vi "Acquisition Message Loop.vi"(8 "error in (no error)":errorcluster, 11 "Message Queues":T2) -> (0 "error out":errorcluster)   [LabVIEW 2024, in "Acquisition.lvlib"]
doc: "Message loop for handling messages pertaining to the acquisition of data from the hardware."
uses:
  Acquisition.lvlib
  <vilib>/Utility/error.llb/Error Cluster From Error Code.vi
  Hardware Configuration.ctl
  support/Message Queue/Message Queue.lvlib
  support/Message Queue/Enqueue Message (Single).vi
  <vilib>/ErrorRing/Error Ring.xnode
  Acquisition State.ctl
  support/Message Queue/Enqueue Message (Array).vi
  support/Message Queue/Message Cluster.ctl
  support/Message Queue/All Message Queues.ctl
  controls/dataRefs.ctl
panel:
  in  "dataRef":T1
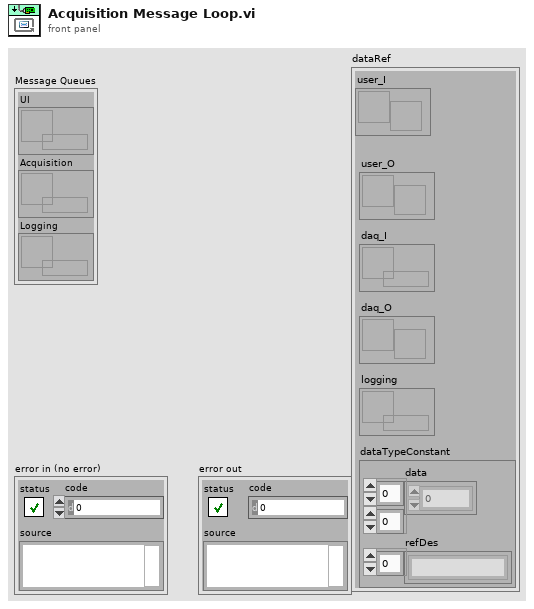
[diagram p1: front panel]
types:
  T1 = typedef "dataRefs.ctl" = cluster{"dataTypeConstant":cluster{"data":dbl[][], "refDes":string[]}, "user_I":refnum<notifier>, "user_O":refnum<notifier>, "daq_O":refnum<notifier>, "logging":refnum<queue>, "daq_I":refnum<queue>}
  T2 = typedef "Message Queue.lvlib/All Message Queues.ctl" = cluster{"UI":refnum<queue>, "Acquisition":refnum<queue>, "Logging":refnum<queue>}
  T3 = typedef "Acquisition.lvlib/Hardware Configuration.ctl" = cluster{"AI":cluster{"DAQmx Channel":tag, "Max Input":dbl, "Min Input":dbl, "Sample Rate":dbl, "DAQmx Task":refnum<k21>, "shunt resistor location":i32, "external shunt resistor value":dbl}, "AO":cluster{"DAQmx Channel":tag, "Max Output":dbl, "Min Output":dbl, "Sample Rate":dbl, "DAQmx Task":refnum<k21>}, "DO":cluster{"DAQmx Channel":tag, "Sample Rate":dbl, "DAQmx Task":refnum<k21>}, "DI":cluster{"DAQmx Channel":tag, "Sample Rate":dbl, "DAQmx Task":refnum<k21>}, "TC":cluster{"DAQmx Channel":tag, "Max Inout":dbl, "Min Input":dbl, "Sample Rate":dbl, "DAQmx Task":refnum<k21>, "resistance configuration":i32, "r0":dbl, "current excitation value":dbl, "current excitation source":i32, "rtd type":i32}}
  T4 = typedef "Acquisition.lvlib/Acquisition State.ctl" = enum16{"Idle", "Acquiring"}
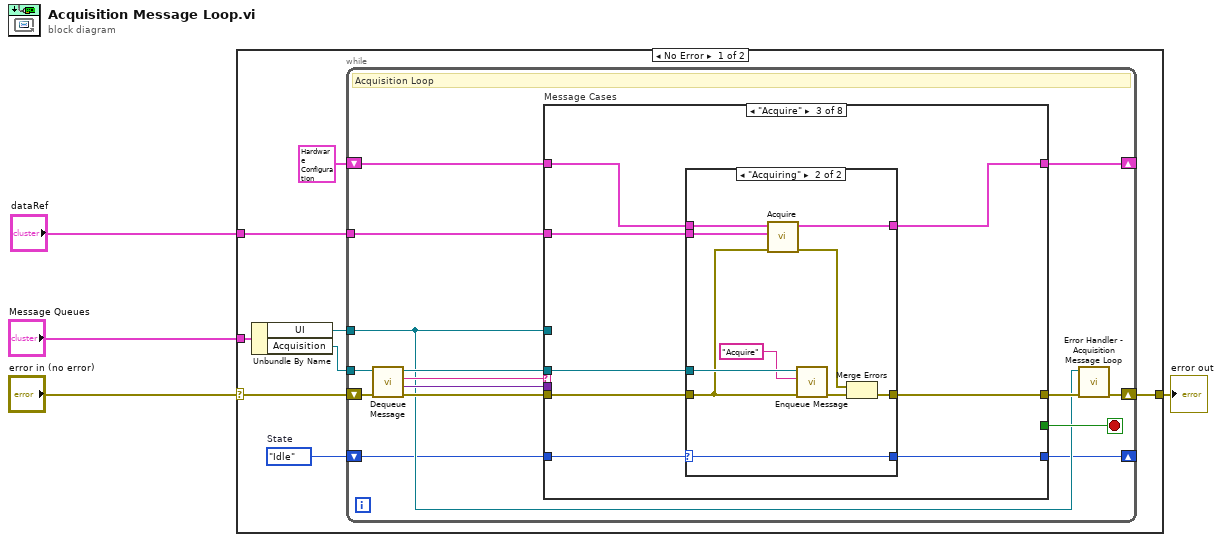
[diagram p0: block diagram]
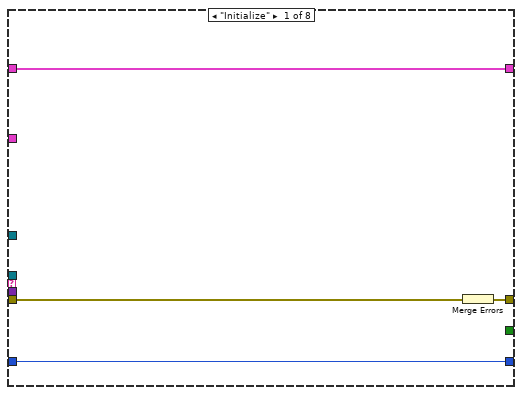
[diagram p2: hidden frame]
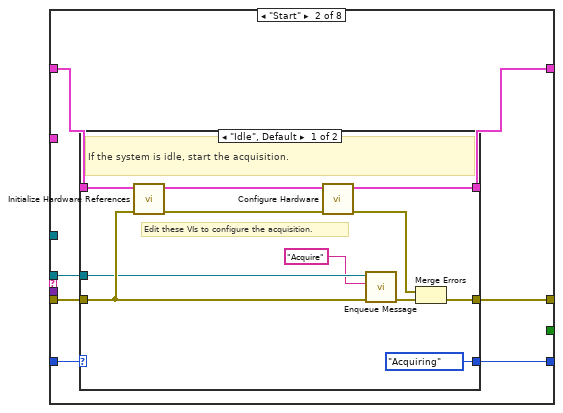
[diagram p3: hidden frame]
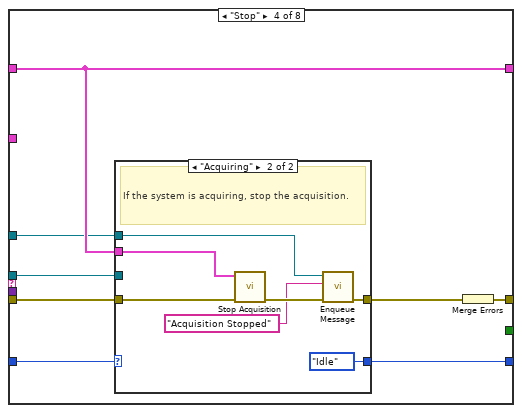
[diagram p6: hidden frame]
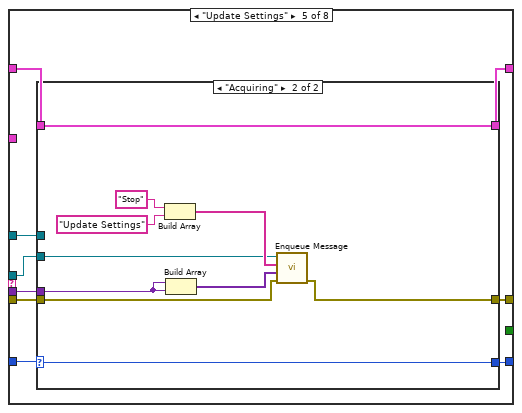
[diagram p8: hidden frame]
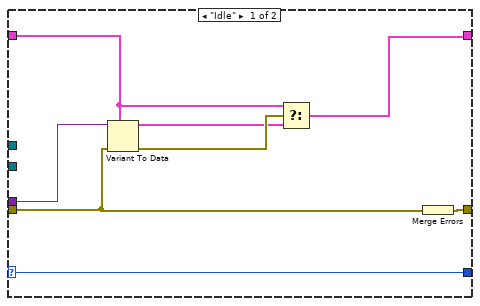
[diagram p9: hidden frame]
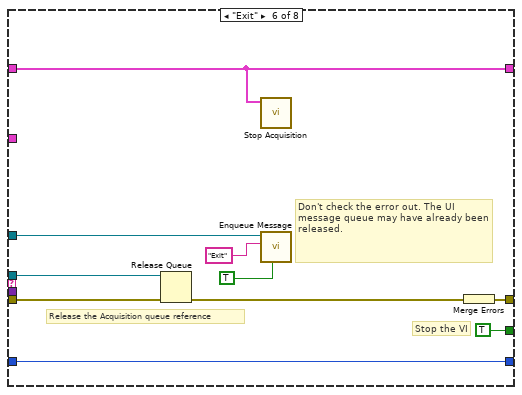
[diagram p10: hidden frame]
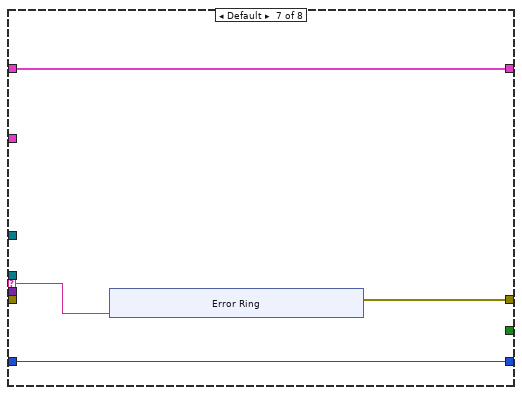
[diagram p11: hidden frame]
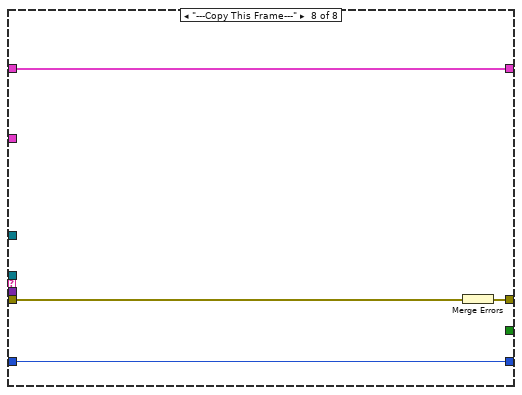
[diagram p12: hidden frame]
diagram:
  n1 = case shown="No Error" "error in (no error)" {
    selector: "error in (no error)" -> [w8 w143]
    tunnel: "Message Queues" -> [w12 _]
    tunnel: [w10 w143] -> w3
    tunnel: "dataRef" -> [w5 _]
    frame No Error {
      w6 = Acquisition_State."Idle"  # State
      n2 = Unbundle By Name(w12) -> ("UI"=w7:refnum<queue>, "Acquisition"=w11:refnum<queue>)
      n3 = while {
        tunnel: w11 -> [w19]
        shift-right: [w26] -> _
        shift-left: T3 {"AI"={"DAQmx Channel"="", "Max Input"=0.0, "Min Input"=0.0, "Sample Rate"=0.0, "DAQmx Task"="", "shunt resistor location"=-1, "external shunt resistor value"=249.0}, "AO"={"DAQmx Channel"="", "Max Output"=0.0, "Min Output"=0.0, "Sample Rate"=0.0, "DAQmx Task"=""}, "DO"={"DAQmx Channel"="", "Sample Rate"=0.0, "DAQmx Task"=""}, "DI"={"DAQmx Channel"="", "Sample Rate"=0.0, "DAQmx Task"=""}, "TC"={"DAQmx Channel"="", "Max Inout"=0.0, "Min Input"=0.0, "Sample Rate"=0.0, "DAQmx Task"="", "resistance configuration"=4, "r0"=100.0, "current excitation value"=0.0025, "current excitation source"=10167, "rtd type"=12481}} ("Data Cluster") -> [w27]
        shift-right: [w17] -> w10
        shift-left: w8 -> [w24]
        tunnel: w7 -> [w16]
        shift-right: [w14] -> _
        shift-left: w6 -> [w15]
        tunnel: w5 -> [w13]
        stop <- w25 stop-if-true
        # "Acquisition Loop"
        n4 = call "Dequeue Message.vi"("error in (no error)"=w24, "Message Queue"=w19) -> ("error out"=w23:errorcluster, "Message Data"=w21:variant, "Message"=w22:string, "dup Message Queue"=w20:refnum<queue>)  [unwired: 6 in]
        n5 = case "Message Cases" shown="\"Acquire\"" w22 {
          selector: w22 -> [_ _ _ _ _ _ w130 _]
          tunnel: w20 -> [_ w35 w59 w78 w91 w120 _ _]
          tunnel: w23 -> [w30 w36 w58 w80 w95 w124 _ w142]
          tunnel: [w31 w38 w60 w81 w99 w126 w129 w140] -> w18
          tunnel: w27 -> [w29 w37 w56 w79 w97 w119 w131 w141]
          tunnel: [w29 w34 w57 w79 w96 w119 w131 w141] -> w26
          tunnel: [_ _ _ _ _ TRUE _ _] -> w25
          tunnel: w21 -> [_ _ _ _ w98 _ _ _]
          tunnel: w16 -> [_ _ _ w77 w92 w125 _ _]
          tunnel: w15 -> [w28 w33 w55 w76 w94 w118 w128 w139]
          tunnel: [w28 w32 w54 w75 w93 w118 w128 w139] -> w14
          tunnel: w13 -> [_ _ w53 _ _ _ _ _]
          frame "Initialize" {
            # "Initialize  - Initialize is currently a no-op.  The hardware initialization takes place in the 'Start' message."
            n6 = Merge Errors(w30) -> (w31:errorcluster)
          }
          frame "Start" {
            # "Start - Configure and start the acquisition."
            n7 = case shown="\"Idle\", Default" w33 {
              selector: w33 -> [_ w50]
              tunnel: [w49 w52] -> w38
              tunnel: w37 -> [w48 w51]
              tunnel: w36 -> [w47 w52]
              tunnel: w35 -> [w45 _]
              tunnel: [w41 w51] -> w34
              tunnel: [Acquisition_State."Acquiring" ("State") w50] -> w32
              frame "Idle", Default {
                # "Edit these VIs to configure the acquisition."
                # "If the system is idle, start the acquisition."
                n8 = call "Initialize Hardware References.vi"("error in (no error)"=w47, "Hardware Resources in"=w48) -> ("error out"=w44:errorcluster, "Hardware Resources out"=w42:T3)  [unwired: 8 in]
                n9 = call "Configure Hardware.vi"("error in (no error)"=w44, "Hardware Resources in"=w42) -> ("error out"=w43:errorcluster, "Hardware Resources out"=w41:T3)  [unwired: 8 in]
                n10 = call-poly "Enqueue Message.vi"("error in (no error)"=w47, "Message"="Acquire", "Message Queue"=w45) -> ("error out"=w46:errorcluster)  [unwired: 7 in, 1 out]
                n11 = Merge Errors(w43, w46) -> (w49:errorcluster)
              }
              frame "Acquiring" {
                # "The system is already acquiring. Ignore the \"Start\" message."
              }
            }
          }
          frame "Acquire" {
            # "Acquire - Acquire data from the hardware. Since this is a continuous acquisition, this message will always message itself to run again."
            n12 = case shown="\"Acquiring\"" w55 {
              selector: w55 -> [w61 w66]
              tunnel: [w62 w73] -> w60
              tunnel: w59 -> [_ w71]
              tunnel: w58 -> [w62 w65]
              tunnel: [w63 w69] -> w57
              tunnel: w56 -> [w63 w68]
              tunnel: [w61 w66] -> w54
              tunnel: w53 -> [_ w64]
              frame "Idle", Default {
              }
              frame "Acquiring" {
                n13 = call "Acquire.vi"("error in (no error)"=w65, "dataRef"=w64, "Hardware Resources in"=w68) -> ("error out"=w70:errorcluster, "Hardware Resources out"=w69:T3)  [unwired: 7 in]
                n14 = call-poly "Enqueue Message.vi"("error in (no error)"=w65, "Message"="Acquire", "Message Queue"=w71) -> ("error out"=w72:errorcluster)  [unwired: 7 in, 1 out]
                n15 = Merge Errors(w70, w72) -> (w73:errorcluster)
              }
            }
          }
          frame "Stop" {
            # "Stop - Stop the Acquisition. Also flush the queue of any pending \"Acquire\" messages."
            n16 = case shown="\"Acquiring\"" w76 {
              selector: w76 -> [w83 _]
              tunnel: w80 -> [w82 w84]
              tunnel: w79 -> [_ w90]
              tunnel: w78 -> [_ _]
              tunnel: w77 -> [_ w89]
              tunnel: [w83 Acquisition_State."Idle" ("State")] -> w75
              tunnel: [w82 w87] -> w74
              frame "Idle", Default {
                # "The system is already idle. Ignore the \"Stop\" message."
              }
              frame "Acquiring" {
                # "If the system is acquiring, stop the acquisition."
                n17 = call "Stop Acquisition.vi"("error in (no error)"=w84, "Hardware Resources in"=w90) -> ("error out"=w88:errorcluster)  [unwired: 9 in]
                n18 = call-poly "Enqueue Message.vi"("error in (no error)"=w88, "Message"="Acquisition Stopped", "Message Queue"=w89) -> ("error out"=w87:errorcluster)  [unwired: 7 in, 1 out]
              }
            }
            n19 = Merge Errors(w74) -> (w81:errorcluster)
          }
          frame "Update Settings" {
            # "New settings are available, update the current ones stored in the shift register with the settings sent as part of the message"
            n20 = case shown="\"Acquiring\"" w94 {
              selector: w94 -> [w100 w116]
              tunnel: [w107 w109] -> w99
              tunnel: w98 -> [w106 w112]
              tunnel: w97 -> [w103 w117]
              tunnel: [w102 w117] -> w96
              tunnel: w95 -> [w101 w110]
              tunnel: [w100 w116] -> w93
              tunnel: w92 -> [_ _]
              tunnel: w91 -> [_ w108]
              frame "Idle" {
                n21 = Variant To Data(error in=w101, type=w103, Variant=w106) -> (data=w104:T3, error out=w105:errorcluster)
                n22 = Select(t=w103, s=w105, f=w104) -> (s? t:f=w102:T3)
                n23 = Merge Errors(w101) -> (w107:errorcluster)
              }
              frame "Acquiring" {
                n24 = Build Array("Stop", "Update Settings") -> (w113:string[])
                n25 = Build Array(w112, w112) -> (w111:variant[])
                n26 = call-poly "Enqueue Message.vi"("error in (no error)"=w110, "Message Data Array"=w111, "Message Array"=w113, "Message Queue"=w108) -> ("error out"=w109:errorcluster)  [unwired: 6 in, 1 out]
              }
            }
          }
          frame "Exit" {
            # "Don't check the error out. The UI message queue may have already been released."
            # "Release the Acquisition queue reference"
            # "Stop the VI"
            # "Exit - Send the Exit message to the UI Message Handler."
            n27 = Release Queue(queue=w120, error in (no error)=w124) -> (error out=w121:errorcluster)  [unwired: 1 in, 2 out]
            n28 = call "Stop Acquisition.vi"("Hardware Resources in"=w119) -> ()  [unwired: 10 in, 1 out]
            n29 = call-poly "Enqueue Message.vi"("Priority Message? (F)"=TRUE, "Message"="Exit", "Message Queue"=w125) -> ()  [unwired: 7 in, 2 out]
            n30 = Merge Errors(w121) -> (w126:errorcluster)
          }
          frame Default {
            # "'Default' case only runs if there is a message that isn't defined in any of the other cases.  Output a programming error."
            n31 = xnode "Error Ring"("parameter 0"=w130) -> ("error out"=w129:errorcluster)
          }
          frame "---Copy This Frame---" {
            # "Duplicate this frame when creating new messages.  Change this comment in the duplicated frame to describe this message."
            n32 = Merge Errors(w142) -> (w140:errorcluster)
          }
        }
        n33 = call "Error Handler - Acquisition Message Loop.vi"("error in (no error)"=w18, "Message Queue"=w16) -> ("dup error in"=w17:errorcluster)  [unwired: 8 in, 1 out]
      }
    }
    frame Error {
    }
  }
  "error out" <- w3
